vi "standby.vi"(8 "error in (no error)":errorcluster, 9 "Parameters":T1, 10 "Model in":refnum<class "Model.lvclass">, 11 "DisabledState in":refnum<class "DisabledState.lvclass">) -> (0 "error out":errorcluster, 2 "Model out":refnum<class "Model.lvclass">, 3 "DisabledState out":refnum<class "DisabledState.lvclass">)   [LabVIEW 2016, in "DisabledState.lvclass"]
uses:
  DisabledState.lvclass
  Model/Model.lvclass
  DataTypes/Topics/CommandStandby.ctl
  DataTypes/Topics/Parts/CommandId.ctl
  DataTypes/Topics/Parts/DetailedStates.ctl
  DataTypes/Topics/M1M3SupportTopics.lvlib
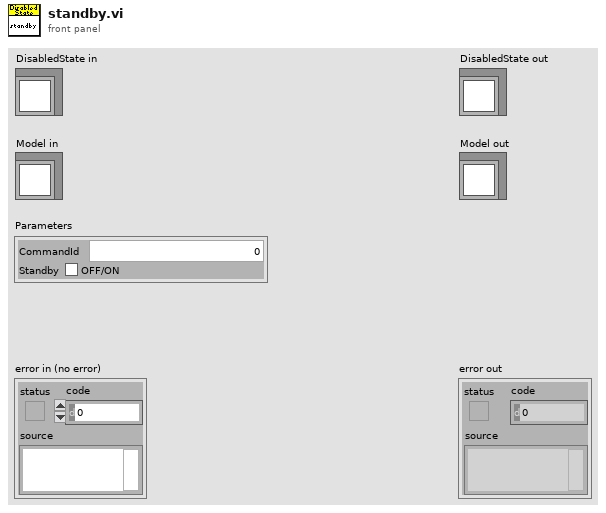
[diagram p1: front panel]
types:
  T1 = typedef "M1M3SupportTopics.lvlib/CommandStandby.ctl" = cluster{"CommandId":T2, "Standby":bool}
  T2 = typedef "M1M3SupportTopics.lvlib/CommandId.ctl" = i32
  T3 = typedef "M1M3SupportTopics.lvlib/DetailedStates.ctl" = enum16{"OfflineState", "InitialState", "StandbyState", "DisabledState", "ParkedState", "FaultState", "ParkedMaintenanceState", "ActiveMaintenanceState"}
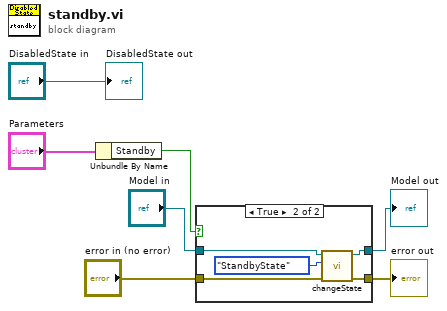
[diagram p0: block diagram]
diagram:
  n1 = Unbundle By Name("Parameters") -> ("Standby"=w1:bool)
  n2 = case shown="True" w1 {
    tunnel: "Model in" -> [w9 w14]
    tunnel: [w9 w12] -> w6
    tunnel: "error in (no error)" -> [w8 w11]
    tunnel: [w8 w10] -> w4
    frame False {
    }
    frame True {
      n3 = call "changeState.vi"("error in (no error)"=w11, "DetailedStates"=DetailedStates."StandbyState", "Model in"=w14) -> ("error out"=w10:errorcluster, "Model out"=w12:refnum<class "Model.lvclass">)  [unwired: 7 in]
    }
  }
  "error out" <- w4
  "Model out" <- w6
  "DisabledState out" <- "DisabledState in"
